vi "Master_Navigator.vi"(10 "velocity from motor Controller":dbl, 11 "x acceleration (g)":dbl) -> (3 "Distance Out":dbl)   [LabVIEW 2018]
uses:
  <vilib>/Analysis/NI_AALPro.lvlib
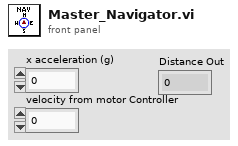
[diagram p1: front panel]
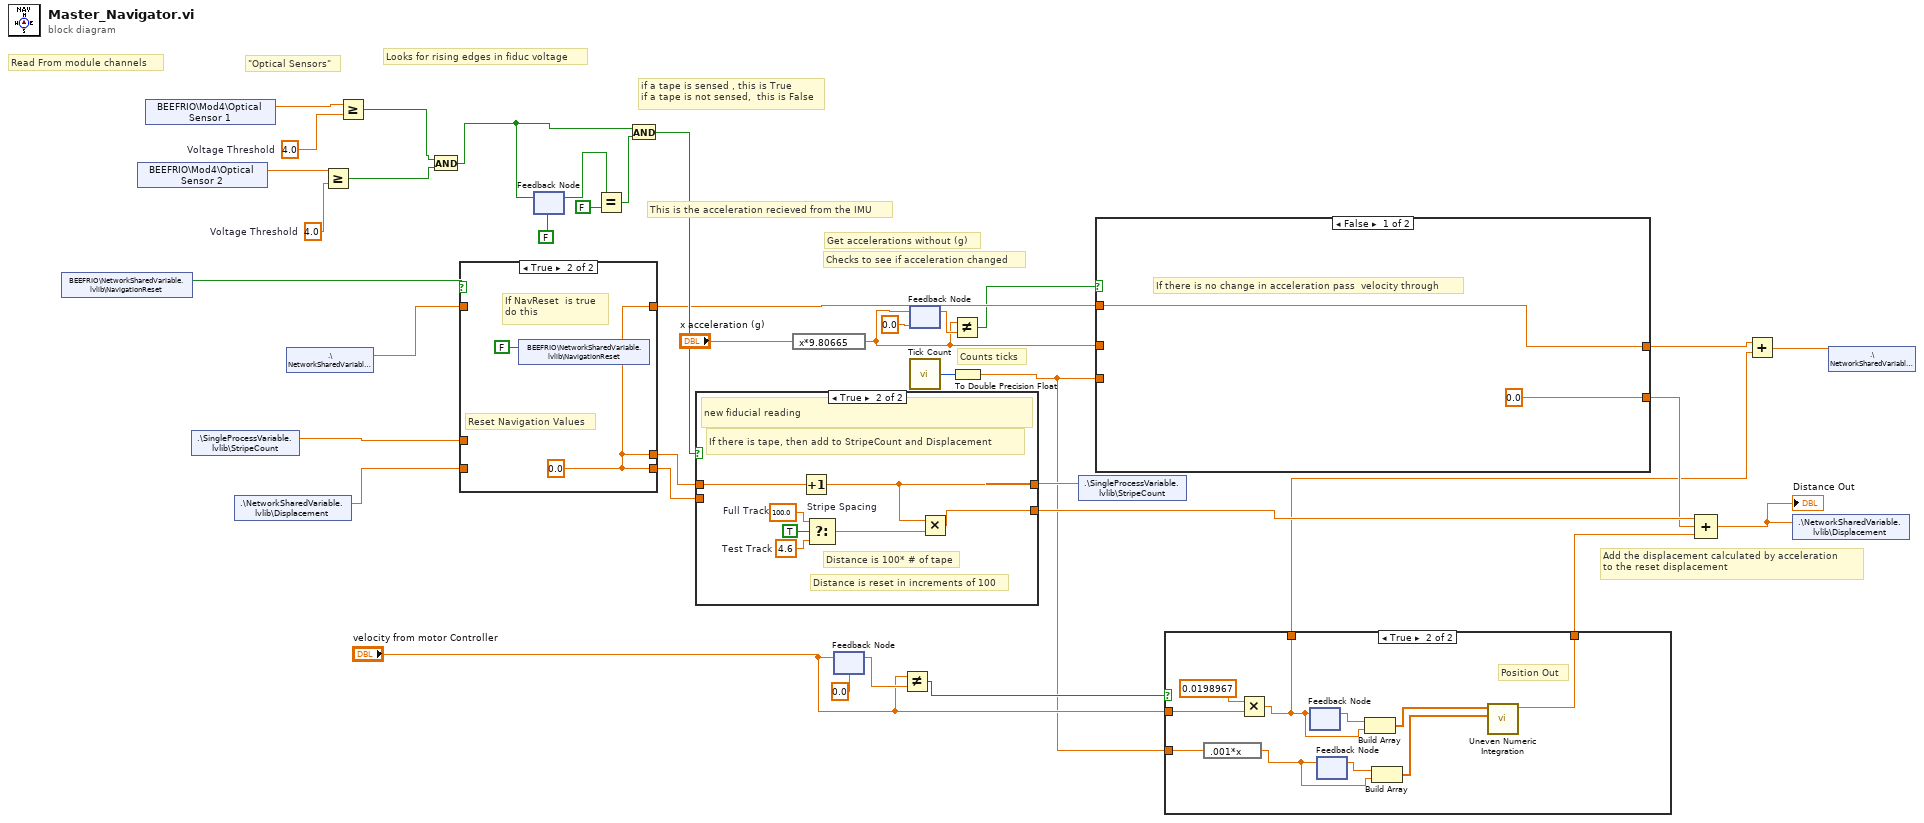
[diagram p0: block diagram]
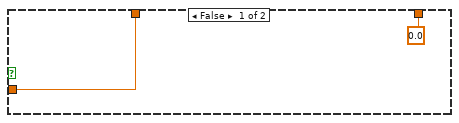
[diagram p2: hidden frame]
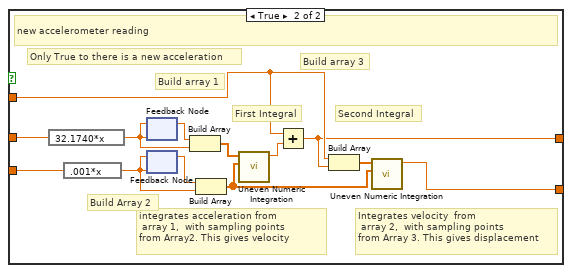
[diagram p4: hidden frame]
diagram:
  w14 = 4.0  # Voltage Threshold
  w37 = 4.0  # Voltage Threshold
  # "This is the acceleration recieved from the IMU"
  # "Counts ticks"
  # "Checks to see if acceleration changed"
  # "Add the displacement calculated by acceleration \nto the reset displacement"
  # "Get accelerations without (g)"
  # "if a tape is sensed , this is True\nif a tape is not sensed,  this is False"
  # "\"Optical Sensors\""
  # "Read From module channels"
  # "Looks for rising edges in fiduc voltage"
  n1 = shared-variable "BEEFRIO\\NetworkSharedVariable.lvlib\\NavigationReset"() -> (w15:bool)  [unwired: 1 in, 1 out]
  n2 = shared-variable "BEEFRIO\\Mod4\\Optical Sensor 2"() -> (w13:dbl)  [unwired: 1 in, 1 out]
  n3 = shared-variable "BEEFRIO\\Mod4\\Optical Sensor 1"() -> (w38:dbl)  [unwired: 1 in, 1 out]
  n4 = shared-variable ".\\SingleProcessVariable.lvlib\\StripeCount"() -> (w30:dbl)  [unwired: 1 in, 1 out]
  n5 = shared-variable ".\\NetworkSharedVariable.lvlib\\Displacement"() -> (w28:dbl)  [unwired: 1 in, 1 out]
  n6 = shared-variable ".\\NetworkSharedVariable.lvlib\\Velocity"() -> (w27:dbl)  [unwired: 1 in, 1 out]
  n7 = Greater Or Equal?(x=w13, y=w14) -> (x >= y?=w11:bool)
  n8 = Greater Or Equal?(x=w38, y=w37) -> (x >= y?=w12:bool)
  n9 = And(x=w12, y=w11) -> (x .and. y?=w10:bool)
  n10 = case shown="True" w15 {
    tunnel: w30 -> [w41 _]
    tunnel: [w41 w42] -> w31
    tunnel: [w40 w42] -> w19
    tunnel: w28 -> [w40 _]
    tunnel: w27 -> [w39 _]
    tunnel: [w39 w42] -> w29
    frame False {
      # "if NavReset  is false\npass data through"
    }
    frame True {
      w42 = 0.0
      # "Reset Navigation Values"
      # "If NavReset  is true\ndo this"
      n11 = shared-variable "BEEFRIO\\NetworkSharedVariable.lvlib\\NavigationReset"(FALSE ("NavReset")) -> ()  [unwired: 1 in, 1 out]
    }
  }
  n12 = feedback-in #1(w10) -> ()
  n13 = feedback #1(FALSE) -> (w33:bool)
  n14 = Equal?(x=w33, y=FALSE) -> (x = y?=w34:bool)
  n15 = And(x=w10, y=w34) -> (x .and. y?=w32:bool)
  n16 = case shown="True" w32 {
    tunnel: [w45 w50] -> w22
    tunnel: w31 -> [w45 w52]
    tunnel: [w44 w51] -> w17
    tunnel: w19 -> [w44 _]
    frame False {
      # "If there is no new tape pass value through"
    }
    frame True {
      w49 = 4.6  # Test Track
      w48 = 100.0  # Full Track
      # "Distance is reset in increments of 100"
      # "Distance is 100* # of tape"
      # "If there is tape, then add to StripeCount and Displacement"
      # "new fiducial reading"
      n17 = Increment(x=w52) -> (x+1=w50:dbl)
      n18 = Select "Stripe Spacing"(t=w48, s=TRUE, f=w49) -> (s? t:f=w47:dbl)
      n19 = Multiply(x=w50, y=w47) -> (x*y=w51:dbl)
    }
  }
  n20 = expression code="x*9.80665"("x acceleration (g)") -> (w21:dbl)
  n21 = feedback-in #2("velocity from motor Controller") -> ()
  n22 = feedback #2(0.0 ("velocity from motor Controller")) -> (w9:dbl)
  n23 = Not Equal?(x="velocity from motor Controller", y=w9) -> (x != y?=w7:bool)
  n24 = feedback-in #3(w21) -> ()
  n25 = feedback #3(0.0 ("x acceleration (g)")) -> (w24:dbl)
  n26 = call "Tick Count"() -> ("Tick Count(mSec)"=w26:u32)
  n27 = Not Equal?(x=w21, y=w24) -> (x != y?=w23:bool)
  n28 = To Double Precision Float(number=w26) -> (double precision float=w5:dbl)
  n29 = shared-variable ".\\SingleProcessVariable.lvlib\\StripeCount"(w22) -> ()  [unwired: 1 in, 1 out]
  n30 = case shown="False" w23 {
    tunnel: w29 -> [w54 w59]
    tunnel: [w54 w58] -> w2
    tunnel: w5 -> [_ w57]
    tunnel: w21 -> [_ w56]
    tunnel: [0.0 ("result") w55] -> w16
    frame False {
      # "If there is no change in acceleration pass  velocity through"
    }
    frame True {
      # "Integrates velocity  from\n array 2,  with sampling points \nfrom Array 3. This gives displacement"
      # "Build array 3"
      # "integrates acceleration from\n array 1,  with sampling points \nfrom Array2. This gives velocity"
      # "Build array 1"
      # "Build Array 2"
      # "Only True to there is a new acceleration"
      # "Second Integral"
      # "First Integral"
      # "new accelerometer reading"
      n31 = expression code="32.1740*x"(w56) -> (w65:dbl)
      n32 = expression code=".001*x"(w57) -> (w66:dbl)
      n33 = feedback #4(w65) -> (w64:dbl)
      n34 = feedback-in #4(w65) -> ()
      n35 = feedback #5(w66) -> (w60:dbl)
      n36 = feedback-in #5(w66) -> ()
      n37 = Build Array(w64, w65) -> (w61:dbl[])
      n38 = Build Array(w60, w66) -> (w63:dbl[])
      n39 = call <vilib>:"Uneven Numeric Integration.vi"("T"=w63, "X"=w61) -> ("result"=w67:dbl)  [unwired: 8 in, 1 out]
      n40 = Add(x=w59, y=w67) -> (x+y=w58:dbl)
      n41 = Build Array(w59, w58) -> (w62:dbl[])
      n42 = call <vilib>:"Uneven Numeric Integration.vi"("T"=w63, "X"=w62) -> ("result"=w55:dbl)  [unwired: 8 in, 1 out]
    }
  }
  n43 = case shown="True" w7 {
    tunnel: "velocity from motor Controller" -> [w69 w79]
    tunnel: w5 -> [_ w75]
    tunnel: [0.0 ("result") w71] -> w4
    tunnel: [w69 w70] -> w1
    frame False {
    }
    frame True {
      # "Position Out"
      n44 = expression code=".001*x"(w75) -> (w73:dbl)
      n45 = Multiply(x=0.0198967, y=w79) -> (x*y=w70:dbl)
      n46 = feedback #6() -> (w77:dbl)  [unwired: 1 in]
      n47 = feedback-in #6(w70) -> ()
      n48 = feedback #7() -> (w74:dbl)  [unwired: 1 in]
      n49 = feedback-in #7(w73) -> ()
      n50 = Build Array(w77, w70) -> (w76:dbl[])
      n51 = Build Array(w74, w73) -> (w72:dbl[])
      n52 = call <vilib>:"Uneven Numeric Integration.vi"("T"=w72, "X"=w76) -> ("result"=w71:dbl)  [unwired: 8 in, 1 out]
    }
  }
  n53 = Compound Arithmetic op=ADD(w17, w16, w4) -> (w18:dbl)
  "Distance Out" <- w18
  n54 = Add(x=w2, y=w1) -> (x+y=w3:dbl)
  n55 = shared-variable ".\\NetworkSharedVariable.lvlib\\Displacement"(w18) -> ()  [unwired: 1 in, 1 out]
  n56 = shared-variable ".\\NetworkSharedVariable.lvlib\\Velocity"(w3) -> ()  [unwired: 1 in, 1 out]
